vi "RSZVB Get Calibration Power Generator Offset.vi"(7 "Generator Number (1)":i32=1, 8 "error in (no error)":errorcluster {"code" format="%.0x"}, 9 "Port Number (1)":i32=1, 10 "Channel (1)":i32=1, 11 "VISA session":refnum<visa-resource-name>) -> (0 "error out":errorcluster {"code" format="%.0x"}, 1 "Cal Power Generator Offset":dbl format="%^.3e", 3 "dup VISA session":refnum<visa-resource-name>)   [LabVIEW 2011]
doc: "This VI returns a gain (positive values) or an attenuation (negative values) in the signal path between the external generator and the calibrated reference plane.\n\nNote(s):\n\n(1) This VI is availble only with R&S ZVA and ZVT instruments. \n\nRemote-control command(s):\nSOURce<Ch>:POWer<Pt>:CORRection:GENerator<Gen>:LEVel:OFFSet?"
uses:
  _utility/RSZVB Global Data.vi
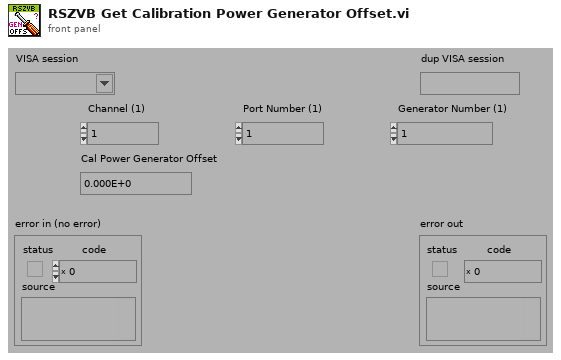
[diagram p1: front panel]
types:
  T1 = cluster{"Error Checking (T: On)":bool, "Installed Options":string[], "Data Valid?":bool, "Ports":i32, "Model":string[], "Option Checking (T: On)":bool}[]
  T2 = cluster{"Error Checking (T: On)":bool, "Installed Options":string[], "Data Valid?":bool, "Ports":i32, "Model":string[], "Option Checking (T: On)":bool}
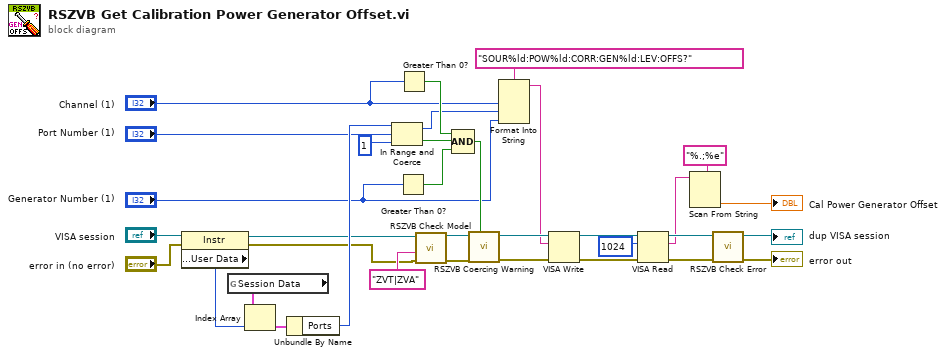
[diagram p0: block diagram]
diagram:
  n1 = property class="Instr"(reference="VISA session", error in="error in (no error)") -> (reference out=w2:refnum<visa-resource-name>, error out=w1:errorcluster, "General Settings:User Data"=w19:u32)
  n2 = global read "RSZVB Global Data.vi" "Session Data"() -> (w20:T1)
  n3 = Index Array(array=w20, index=w19) -> (element=w21:T2)
  n4 = Unbundle By Name(w21) -> ("Ports"=w15:i32)
  n5 = In Range and Coerce(upper limit=w15, x="Port Number (1)", lower limit=1) -> (coerced(x)=w16:i32, In Range?=w17:bool)
  n6 = Greater Than 0?(x="Generator Number (1)") -> (x > 0?=w6:bool)
  n7 = Greater Than 0?(x="Channel (1)") -> (x > 0?=w23:bool)
  n8 = call "RSZVB Check Model.vi"("error in (no error)"=w1, "Model"="ZVT|ZVA" ("Options"), "VISA session"=w2) -> ("error out"=w4:errorcluster, "dup VISA session"=w3:refnum<visa-resource-name>)  [unwired: 7 in]
  n9 = Compound Arithmetic op=AND(w23, w17, w6) -> (w22:bool)
  n10 = call "RSZVB Coercing Warning.vi"("In Range?"=w22, "error in (no error)"=w4, "VISA session"=w3) -> ("error out"=w26:errorcluster, "dup VISA session"=w27:refnum<visa-resource-name>)  [unwired: 7 in]
  n11 = Format Into String(format string="SOUR%ld:POW%ld:CORR:GEN%ld:LEV:OFFS?", "Channel (1)", w16, "Generator Number (1)") -> (resulting string=w24:string)  [unwired: 2 in, 1 out]
  n12 = VISA Write(VISA resource name=w27, write buffer=w24, error in (no error)=w26) -> (VISA resource name out=w28:refnum<visa-resource-name>, error out=w29:errorcluster)  [unwired: 1 out]
  n13 = VISA Read(VISA resource name=w28, byte count=u32 1024 ("byte count (0)"), error in (no error)=w29) -> (VISA resource name out=w33:refnum<visa-resource-name>, read buffer=w30:string, error out=w32:errorcluster)  [unwired: 1 out]
  n14 = Scan From String(format string="%.;%e", input string=w30) -> (output 1=→"Cal Power Generator Offset":dbl)  [unwired: 3 in, 3 out]
  n15 = call "RSZVB Check Error.vi"("error in (no error)"=w32, "VISA session"=w33) -> ("error out"=→"error out":errorcluster, "dup VISA session"=→"dup VISA session":refnum<visa-resource-name>)  [unwired: 8 in]
